vi "Execute.vi"(8 "error in":errorcluster, 10 "Shifted Error in":refnum<class "Error.lvclass">, 11 "ERROR_Stop in":refnum<class "ERROR_Stop.lvclass">) -> (0 "error out":errorcluster, 1 "STOP?":bool, 2 "Shifted Error out":refnum<class "Error.lvclass">, 3 "ERROR_Stop out":refnum<class "ERROR_Stop.lvclass">)   [LabVIEW 2019, in "TSC Error.lvlib" / "ERROR_Stop.lvclass"]
doc: "This VI will set the STOP? Boolean to stop the Error Loop.\n\nInputs:\n-ERROR_Stop in [obj] - the dynamic dispatch input class\n-Shifted Error in [obj] - the shifted error class with shared information\n-error in\n\nOutputs:\n-ERROR_Stop out [obj] - the dynamic dispatch output class\n-Shifted Error in [obj] - the shifted error class with shared information\n-STOP? [Boolean] - the output Boolean used to stop the Error Loop\n-error out\n________________________________________________________________________________\n<b>Code Developed By:</b>\nDaniel Coons\nTechnology Service Corporation\n1983 S Liberty Drive\nBloomington, IN 47403\nPhone: 812 558-7100\ndaniel.coons@tsc.com\nwww.tsc.com\n\n<b>Date Created:</b> 11 AUG 2014\n<b>Date Updated:</b>"
uses:
  ERROR_Stop.lvclass
  Error/Error.lvclass
  TSC Error.lvlib
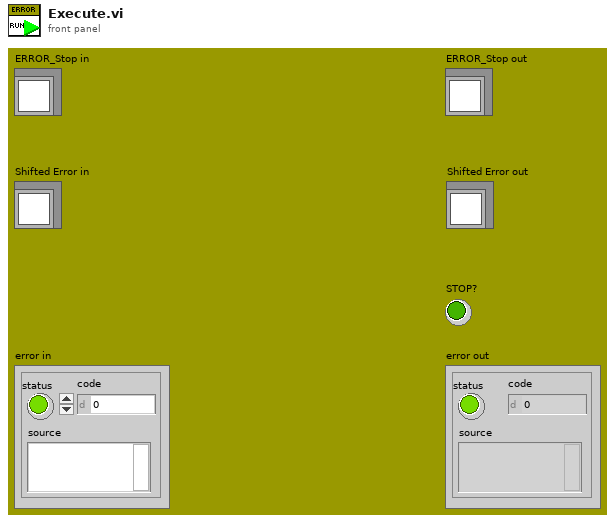
[diagram p1: front panel]
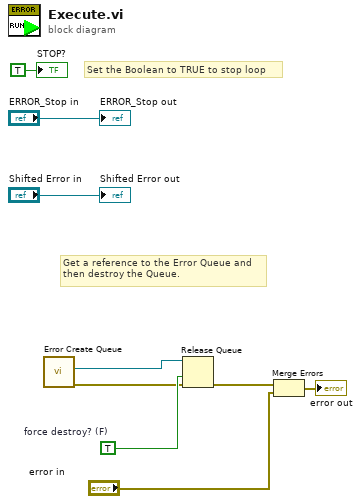
[diagram p0: block diagram]
diagram:
  w6 = TRUE  # force destroy? (F)
  # "Set the Boolean to TRUE to stop loop"
  # "Get a reference to the Error Queue and\nthen destroy the Queue."
  n1 = call "Error Create Queue.vi"() -> ("error out"=w2:errorcluster, "Error Queue out"=w1:refnum<queue>)  [unwired: 9 in, 1 out]
  n2 = Release Queue(queue=w1, force destroy? (F)=w6, error in (no error)=w2) -> (error out=w8:errorcluster)  [unwired: 2 out]
  n3 = Merge Errors(w8, "error in") -> (→"error out":errorcluster)
  "ERROR_Stop out" <- "ERROR_Stop in"
  "STOP?" <- TRUE
  "Shifted Error out" <- "Shifted Error in"
